vi "cropInactive.vi"(2 "Scan in":refnum<class "Scan.lvclass">, 3 "Whole camera frame":u16[][](array[numeric]), 4 "cropLines":i32=1) -> (1 "Cropped camera frame":u16[][](array[numeric]))   [LabVIEW 2017]
uses:
  classes/Scans/Scan.lvclass
  classes/Scans/Scan.lvclass/Scan.ctl
  classes/Scans/Read Total A-scans per frame.vi
panel:
  out "size(s)":i32[](array[numeric])
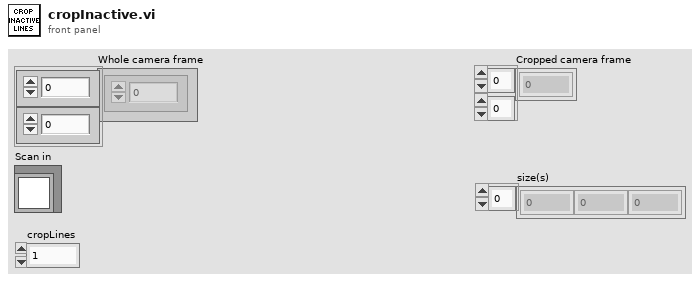
[diagram p1: front panel]
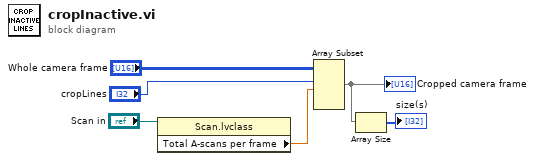
[diagram p0: block diagram]
diagram:
  n1 = property class="Scan.lvclass"(reference="Scan in") -> ("Total A-scans per frame"=w4:dbl)  [unwired: 1 in, 2 out]
  n2 = Array Subset(array="Whole camera frame", index (row)="cropLines", length (row)=w4) -> (w3:u16[][])  [unwired: 2 in]
  "Cropped camera frame" <- w3
  n3 = Array Size(array=w3) -> (size(s)=→"size(s)":i32[])
